vi "IMAQImageTypeToOLV.vi"(8 "error in":errorcluster, 11 "IMAQ Image Type":T1 items=["Grayscale (U8)", "Grayscale (I16)", "Grayscale (SGL)", "Complex (CSG)", "RGB (U32)", "HSL (U32)", "RGB (U64)", "Grayscale (U16)"]) -> (0 "error out":errorcluster, 3 "OLV Image Type":T2)   [LabVIEW 2020, in "OpenLvVision_Image.lvlib" / "Management.lvlib"]
doc: "Convert the OLV image format to the IMAQ image format"
uses:
  Management.lvlib
  TypeDef/ImageType.ctl
  <vilib>/Utility/error.llb/Error Cluster From Error Code.vi
  <vilib>/ErrorRing/Error Ring.xnode
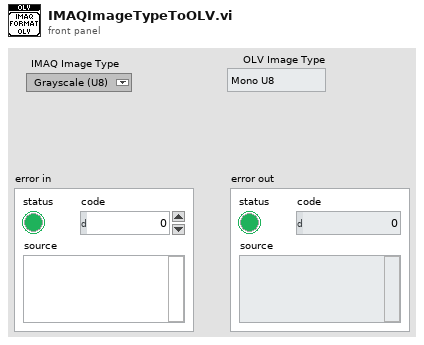
[diagram p1: front panel]
types:
  T1 = typedef "Image Type" = u32
  T2 = typedef "OpenLvVision_Image.lvlib/Management.lvlib/ImageType.ctl" = enum16{"Mono U8", "Mono U16", "Mono I16", "Mono SGL", "Color U32", "Color U64", "Complex SGL"}
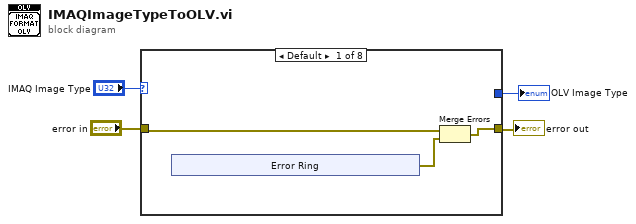
[diagram p0: block diagram]
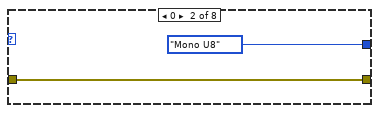
[diagram p2: hidden frame]
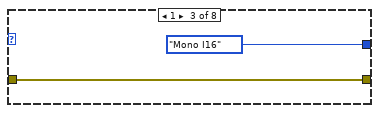
[diagram p3: hidden frame]
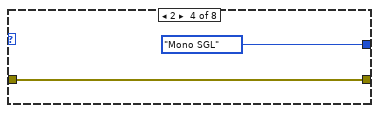
[diagram p4: hidden frame]
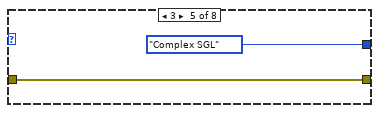
[diagram p5: hidden frame]
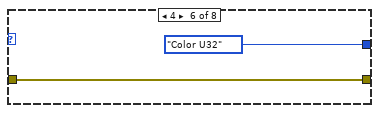
[diagram p6: hidden frame]
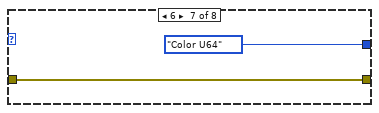
[diagram p7: hidden frame]
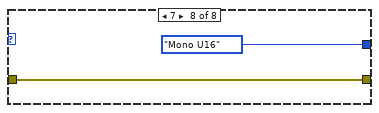
[diagram p8: hidden frame]
diagram:
  n1 = case shown="Default" "IMAQ Image Type" {
    tunnel: [w7 w13 w15 w17 w19 w21 w23 w25] -> w3
    tunnel: "error in" -> [w6 w13 w15 w17 w19 w21 w23 w25]
    tunnel: [_ ImageType."Mono U8" ("OLV Image Type") ImageType."Mono I16" ("OLV Image Type") ImageType."Mono SGL" ("OLV Image Type") ImageType."Complex SGL" ("OLV Image Type") ImageType."Color U32" ("OLV Image Type") ImageType."Color U64" ("OLV Image Type") ImageType."Mono U16" ("OLV Image Type")] -> w1
    frame Default {
      n2 = xnode "Error Ring"() -> ("error out"=w5:errorcluster)
      n3 = Merge Errors(w6, w5) -> (w7:errorcluster)
    }
    frame 0 {
    }
    frame 1 {
    }
    frame 2 {
    }
    frame 3 {
    }
    frame 4 {
    }
    frame 6 {
    }
    frame 7 {
    }
  }
  "OLV Image Type" <- w1
  "error out" <- w3
